vi "Insert Scope Errors.vi"(7 "scope":T1=enum."global", 8 "error in (no error)":errorcluster, 10 "error codes file content":cluster{"properties":T2, "errors":T3[]}[](array[cluster]), 11 "error list <top> in":variant) -> (0 "error out":errorcluster, 3 "error list <top> out":variant)   [LabVIEW 2017]
uses:
  Error Code File Properties.ctl
  Error File Management/Controls/NI Error.ctl
  Scope.ctl
  Error File Management/Error File Management.lvlib
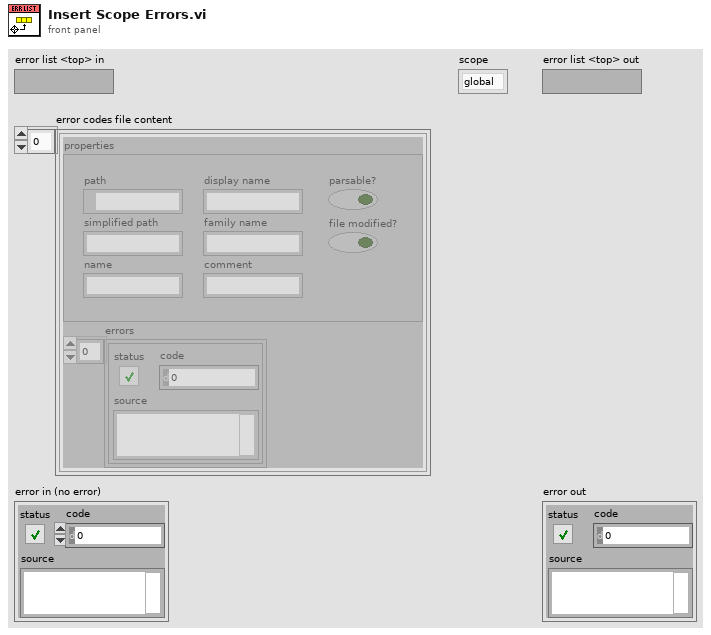
[diagram p1: front panel]
types:
  T1 = typedef "Scope.ctl" = enum16{"project", "global"}
  T2 = typedef "Error Code File Properties.ctl" = cluster{"path":path, "simplified path":string, "name":string, "display name":string, "family name":string, "comment":string, "parsable?":bool, "file modified?":bool}
  T3 = typedef "Error File Management.lvlib/NI Error.ctl" = errorcluster
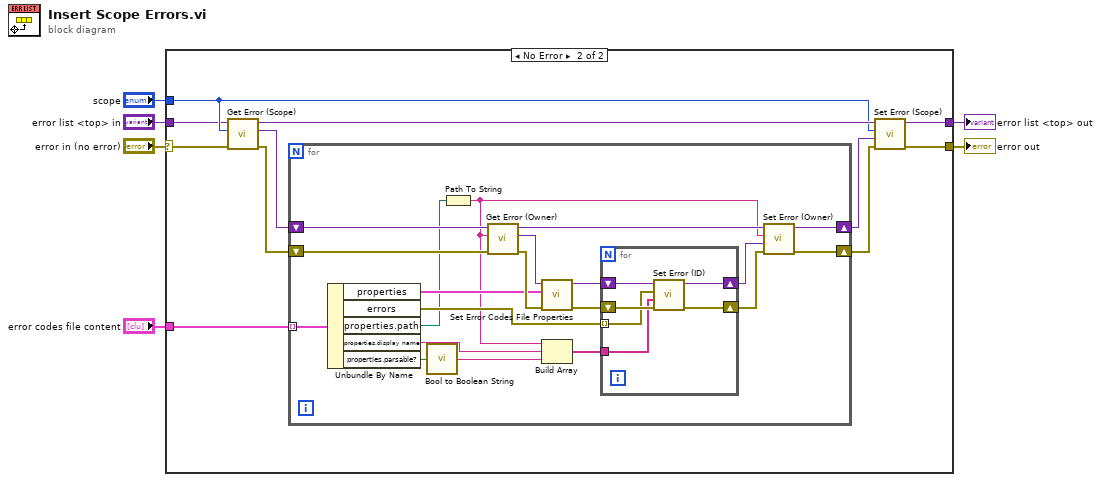
[diagram p0: block diagram]
diagram:
  n1 = case shown="No Error" "error in (no error)" {
    selector: "error in (no error)" -> [w8 w11]
    tunnel: "error codes file content" -> [_ w14]
    tunnel: "scope" -> [_ w13]
    tunnel: [w8 w12] -> w3
    tunnel: "error list <top> in" -> [w7 w10]
    tunnel: [w7 w9] -> w1
    frame Error {
    }
    frame No Error {
      n2 = call "Get Error (Scope).vi"("error in (no error)"=w11, "scope"=w13, "error list <top>"=w10) -> ("error out"=w15:errorcluster, "error list <scope>"=w17:variant, "error list <top> dup"=w16:variant)  [unwired: 5 in, 1 out]
      n3 = for {
        shift-right: [w38] -> w18
        shift-left: w15 -> [w37]
        shift-right: [w39] -> w19
        shift-left: w17 -> [w36]
        tunnel: w14 -> [w28] mode=indexing
        n4 = Unbundle By Name(w28) -> ("properties"=w27:T2, "errors"=w26:T3[], "properties.path"=w25:path, "properties.display name"=w22:string, "properties.parsable?"=w24:bool)
        n5 = call "Bool to Boolean String.vi"("bool"=w24) -> ("boolean string"=w21:string)
        n6 = Path To String(path=w25) -> (string=w23:string)
        n7 = call "Get Error (Owner).vi"("error in (no error)"=w37, "owner"=w23, "error list <scope>"=w36) -> ("error out"=w33:errorcluster, "error list <owner>"=w30:variant, "error list <scope> dup"=w34:variant)  [unwired: 5 in, 1 out]
        n8 = call "Set Error Codes File Properties.vi"("error in (no error)"=w33, "properties"=w27, "error list <owner> in"=w30) -> ("error out"=w31:errorcluster, "error list <owner> out"=w29:variant)  [unwired: 7 in]
        n9 = Build Array(w23, w22, w21) -> (w20:string[])
        n10 = for {
          shift-right: [w43] -> w32
          shift-left: w31 -> [w44]
          shift-right: [w45] -> w35
          shift-left: w29 -> [w42]
          tunnel: w26 -> [w41] mode=indexing
          tunnel: w20 -> [w40]
          n11 = call "Set Error (ID).vi"("error in (no error)"=w44, "attributes"=w40, "new error"=w41, "error list <owner> in"=w42) -> ("error out"=w43:errorcluster, "error list <owner> out"=w45:variant)  [unwired: 6 in]
        }
        n12 = call "Set Error (Owner).vi"("error in (no error)"=w32, "error list <owner>"=w35, "owner"=w23, "error list <scope> in"=w34) -> ("error out"=w38:errorcluster, "error list <scope> out"=w39:variant)  [unwired: 6 in]
      }
      n13 = call "Set Error (Scope).vi"("error in (no error)"=w18, "error list <scope>"=w19, "scope"=w13, "error list <top> in"=w16) -> ("error out"=w12:errorcluster, "error list <top> out"=w9:variant)  [unwired: 6 in]
    }
  }
  "error out" <- w3
  "error list <top> out" <- w1
